vi "Read N channel.vi"(8 "error in (no error)":errorcluster, 11 "MB_v2 in":refnum<class "Modbus Master CR.lvclass">) -> (0 "error out":errorcluster, 2 "N channel":T1, 3 "MB_v2 out":refnum<class "Modbus Master CR.lvclass">)   [LabVIEW 2021, in "Modbus Master CR.lvclass"]
uses:
  Modbus Master CR.lvclass
  ctl/N channel.ctl
  Modbus Master CR.lvclass/Modbus Master CR.ctl
  Data Model/Device Data Model.lvclass
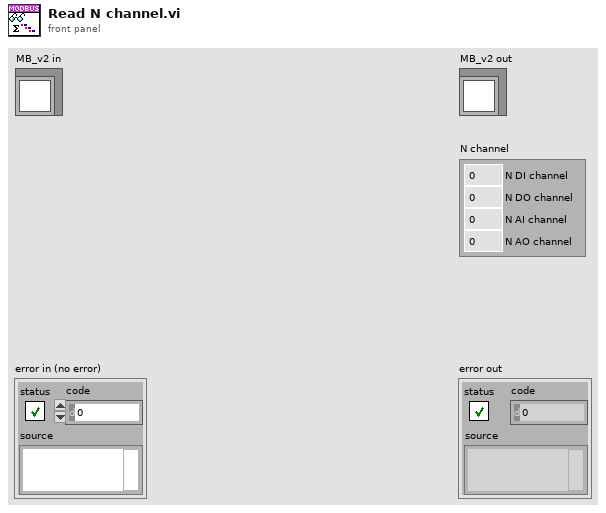
[diagram p1: front panel]
types:
  T1 = typedef "Modbus Master CR.lvclass/N channel.ctl" = cluster{"N DI channel":u16, "N DO channel":u16, "N AI channel":u16, "N AO channel":u16}
  T2 = typedef "Device Data Model.lvclass/N channel.ctl" = cluster{"N DI channel":i32, "N DO channel":i32, "N AI channel":i32, "N AO channel":i32}
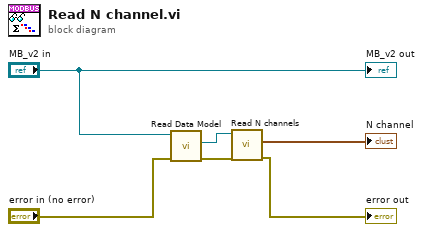
[diagram p0: block diagram]
diagram:
  n1 = call "Read Data Model.vi"("error in (no error)"="error in (no error)", "MB_TCP in"="MB_v2 in") -> ("error out"=w1:errorcluster, "Data Model"=w2:refnum<class "Device Data Model.lvclass">)  [unwired: 7 in, 1 out]
  n2 = call-dynamic "Read N channels.vi"("error in (no error)"=w1, "device data model in"=w2) -> ("error out"=→"error out":errorcluster, "N channel"=→"N channel":T2)  [unwired: 7 in, 1 out]
  "MB_v2 out" <- "MB_v2 in"
